vi "New Reg0Write Command.vi"(0 "RFFE Reg0Write Command in":refnum<class "RFFE Reg0Write Command.lvclass">, 5 "Slave Address":T2=12 format="%02x", 7 "Register Data":T1 format="%02x", 11 "error in (no error)":errorcluster) -> (4 "RFFE Reg0Write Command out":refnum<class "RFFE Reg0Write Command.lvclass">, 15 "error out":errorcluster)   [LabVIEW 2018, in "MIPI RFFE API.lvlib" / "RFFE Reg0Write Command.lvclass"]
uses:
  RFFE Reg0Write Command.lvclass
  C:/Users/semoore/Projects/mipi-rffe-labview-oop/Command/RFFE Command.lvclass
  Slave Address.ctl
  Register Data.ctl
  Register Address.ctl
  RFFE Reg0Write Command.lvclass/RFFE Reg0Write Command.ctl
  Command/RFFE Command.lvclass
  MIPI RFFE API.lvlib
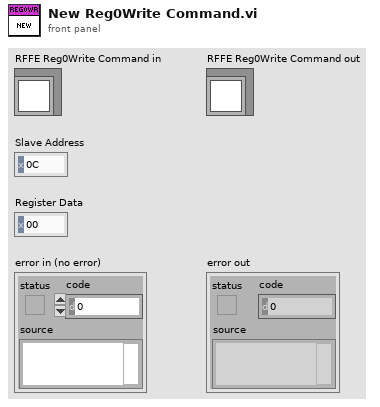
[diagram p1: front panel]
types:
  T1 = typedef "MIPI RFFE API.lvlib/Register Data.ctl" = u8
  T2 = typedef "MIPI RFFE API.lvlib/Slave Address.ctl" = u8
  T3 = typedef "MIPI RFFE API.lvlib/Register Address.ctl" = u16
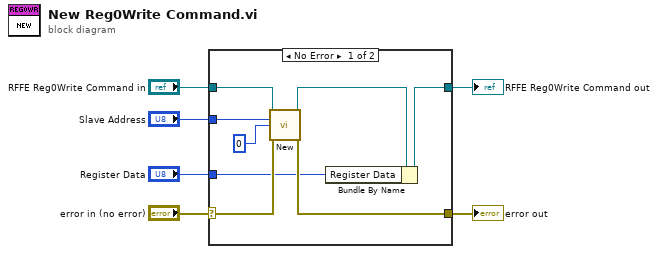
[diagram p0: block diagram]
diagram:
  n1 = case shown="No Error" "error in (no error)" {
    selector: "error in (no error)" -> [w11 w16]
    tunnel: [w10 w16] -> w5
    tunnel: [w14 w15] -> w1
    tunnel: "RFFE Reg0Write Command in" -> [w13 w15]
    tunnel: "Slave Address" -> [w9 _]
    tunnel: "Register Data" -> [w8 _]
    frame No Error {
      n2 = call "New.vi"("RFFE Command in"=w13, "Slave Address"=w9, "Register Address"=T3 0, "error in (no error)"=w11) -> ("RFFE Command out"=w12:refnum<class "RFFE Reg0Write Command.lvclass">, "error out"=w10:errorcluster)  [unwired: 10 in]
      n3 = Bundle By Name(cluster=w12, "Register Data"=w8) -> (w14:refnum<class "RFFE Reg0Write Command.lvclass">)
    }
    frame Error {
    }
  }
  "error out" <- w5
  "RFFE Reg0Write Command out" <- w1
